vi "MT Align To Ideal Symbols (Offset PSK).vi"(0 "input complex waveform":T1={"t0"=0.0, "dt"=1.0, "Y"=[]} {"Y" format="%.3f"; "dt" format="%^.2e"; "t0" format="%.4f"}, 5 "matched filter coefficients":dbl[](array[numeric]) format="%^.2e", 7 "samples per symbol (16)":i32=16, 11 "error in (no error)":errorcluster, 13 "reset? (T)":bool=TRUE) -> (4 "output complex waveform":T1 {"Y" format="%.3f"; "dt" format="%^.2e"; "t0" format="%.4f"}, 6 "output complex waveform (offset removed)":cluster{"t0":dbl, "dt":dbl, "Y":cdb[]}={"t0"=0.0, "dt"=0.25, "Y"=[]}, 8 "waveform alignment offset (samples)":dbl, 15 "error out":errorcluster)   [LabVIEW 2020, in "niDMT.lvlib"]
doc: "This polymorphic instance aligns the first sample of the <B>input complex waveform</B> to the ideal symbol timing instant for an offset PSK (OPSK) modulation scheme. This instance returns an <B>output complex waveform (offset removed) </B> with the 1/2 symbol I/Q offset removed. Wire the <B>output complex waveform (offset removed)</B> to the MT Decimate Oversampled Waveform VI to obtain the demodulated soft symbol decisions."
uses:
  <vilib>/addons/Modulation/niDMT.lvlib
  <vilib>/addons/Modulation/Analog/controls/Complex Data Waveform.ctl
  <vilib>/addons/Modulation/niAMT.lvlib
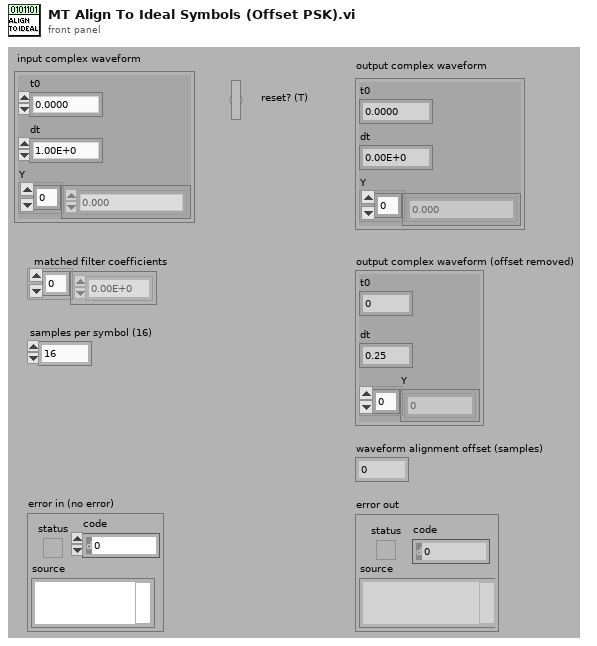
[diagram p1: front panel]
types:
  T1 = typedef "niAMT.lvlib/Complex Data Waveform.ctl" = cluster{"t0":dbl, "dt":dbl, "Y":cdb[]}
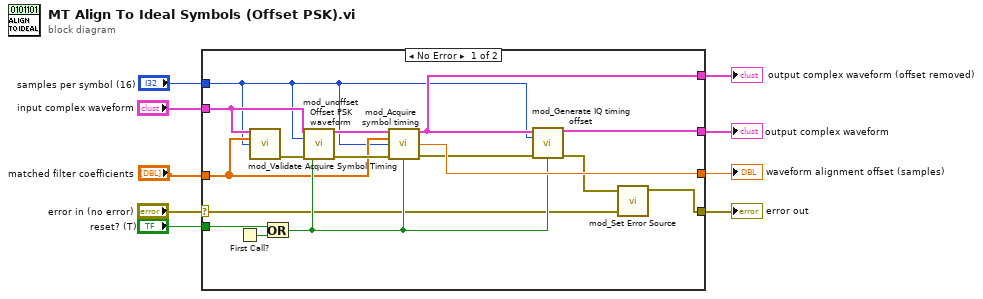
[diagram p0: block diagram]
diagram:
  n1 = case shown="No Error" "error in (no error)" {
    selector: "error in (no error)" -> [w16 w26]
    tunnel: "input complex waveform" -> [w11 _]
    tunnel: "matched filter coefficients" -> [w13 _]
    tunnel: "samples per symbol (16)" -> [w10 _]
    tunnel: "reset? (T)" -> [w25 _]
    tunnel: [w14 w26] -> w4
    tunnel: [w18 _] -> w3
    tunnel: [w23 _] -> w2
    tunnel: [w19 _] -> w1
    frame No Error {
      n2 = First Call?() -> (First Call?: T/F=w24:bool)
      n3 = call <vilib>:"mod_Validate Acquire Symbol Timing.vi"("input complex waveform"=w11, "matched filter coefficients"=w13, "samples per symbol (16)"=w10) -> ("error out"=w12:errorcluster)  [unwired: 12 out]
      n4 = Or(x=w25, y=w24) -> (x .or. y?=w20:bool)
      n5 = call <vilib>:"mod_unoffset Offset PSK waveform.vi"("input complex waveform"=w11, "samples per symbol (16)"=w10, "error in (no error)"=w12, "reset? (T)"=w20) -> ("output complex waveform"=w21:T1, "error out"=w22:errorcluster)  [unwired: 10 out]
      n6 = call <vilib>:"mod_Acquire symbol timing.vi"("input complex waveform"=w21, "matched filter coefficients"=w13, "samples per symbol (16)"=w10, "error in (no error)"=w22, "reset? (T)"=w20) -> ("output complex waveform"=w19:T1, "waveform alignment offset"=w23:dbl, "error out"=w17:errorcluster)  [unwired: 8 out]
      n7 = call <vilib>:"mod_Generate IQ timing offset.vi"("input complex waveform"=w19, "samples per symbol"=w10, "error in (no error)"=w17, "reset? (T)"=w20) -> ("output complex waveform"=w18:T1, "error out"=w15:errorcluster)  [unwired: 10 out]
      n8 = call <vilib>:"mod_Set Error Source.vi"("initial error in (no error)"=w16, "final error in (no error)"=w15) -> ("error out"=w14:errorcluster)  [unwired: 3 out]
    }
    frame Error {
    }
  }
  "error out" <- w4
  "output complex waveform" <- w3
  "waveform alignment offset (samples)" <- w2
  "output complex waveform (offset removed)" <- w1
